vi "RunThis.vi"() -> ()   [LabVIEW 2017]
uses:
  states.ctl
  <vilib>/myRIO/Express VI/Onboard IO/DI/DI Express VI.xnode
  <vilib>/myRIO/Instrument Drivers/Onboard IO/DIO/typedefs/DIO Reference.ctl
  <vilib>/myRIO/Instrument Drivers/Onboard IO/DIO/DIO.lvlib
  <vilib>/myRIO/Common/Instrument Driver Framework/myRIO v1.0/DIO/typedefs/DIO Channels List.ctl
  <vilib>/myRIO/Common/Instrument Driver Framework/myRIO v1.0/DIO/typedefs/DIO Channels Enum.ctl
  <vilib>/myRIO/Common/Instrument Driver Framework/Utilities/typedefs/myRIO Generic Hardware Reference.ctl
  <vilib>/myRIO/Common/Instrument Driver Framework/Utilities/typedefs/myRIO v1.0 Reference.ctl
  <vilib>/myRIO/Common/Instrument Driver Framework/Utilities/typedefs/Generic FPGA Reference.ctl
  <vilib>/myRIO/Common/Instrument Driver Framework/Utilities/typedefs/Hardware Version Enum.ctl
  <vilib>/myRIO/Instrument Drivers/Onboard IO/DIO/vis/Read.vi
  <vilib>/myRIO/Instrument Drivers/Onboard IO/DIO/vis/myRIO DIO Open.xnode
  <vilib>/userdefined/High Color/nirio_resource_hc.ctl
  <vilib>/myRIO/Common/Instrument Driver Framework/myRIO v1.0/DIO/vis/myRIO v1.1 Open DIO.vi
  <vilib>/myRIO/Common/Instrument Driver Framework/Utilities/vis/Is FPGA Ref Available.vi
  encoderposition.ctl
  <vilib>/myRIO/Express VI/Onboard IO/DO/DO Express VI.xnode
  <vilib>/myRIO/Instrument Drivers/Onboard IO/DIO/vis/Write.vi
panel:
  in  "led ms":u32=25
  in  "Motor B":dbl
  out "ride mode duty cycle":dbl format="%.2f"
  out "rps (ride mode)":dbl
  out "Button 4":bool
  out "Counter Value":i32
  out "Button 1":bool
  out "Button 3":bool
  out "Button 2":bool
  in  "Stop Button":bool
  # "Control Panel"
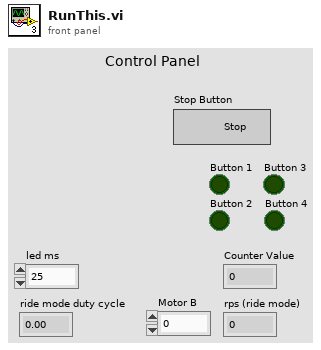
[diagram p1: front panel]
types:
  T1 = typedef "states.ctl" = enum16{"Calibration", "Button Debounce", "Reset Encoder", "Standby", "Go to Horse 1", "Go to Horse 2", "Go to Horse 3", "Go to Horse 4", "Ride Mode"}
  T2 = typedef "DIO.lvlib/DIO Reference.ctl" = cluster{"myRIO Reference":T3, "DIO Channels List":T7}
  T3 = typedef "myRIO Generic Hardware Reference.ctl" = cluster{"myRIO Model":T4, "myRIO Hardware Reference":T5}
  T4 = typedef "Hardware Version Enum.ctl" = enum16{"Unknown", "myRIO-1900", "myRIO-1950", "roboRIO", "NI ELVIS RIO CM"}
  T5 = typedef "myRIO v1.0 Reference.ctl" = cluster{"Generic FPGA Reference":T6, "Allow multiple opens":bool}
  T6 = typedef "Generic FPGA Reference.ctl" = refnum<k20>
  T7 = typedef "DIO Channels List.ctl" = T8[]
  T8 = typedef "DIO Channels Enum.ctl" = enum16{"Not Connected", "C/DIO0", "C/DIO1", "C/DIO2", "C/DIO3", "C/DIO4", "C/DIO5", "C/DIO6", "C/DIO7", "A/DIO0", "A/DIO1", "A/DIO2", "A/DIO3", "A/DIO4", "A/DIO5", "A/DIO6", "A/DIO7", "A/DIO8", "A/DIO9", "A/DIO10", "A/DIO11", "A/DIO12", "A/DIO13", "A/DIO14", "A/DIO15", "B/DIO0", "B/DIO1", "B/DIO2", "B/DIO3", "B/DIO4", "B/DIO5", "B/DIO6", "B/DIO7", "B/DIO8", "B/DIO9", "B/DIO10", "B/DIO11", "B/DIO12", "B/DIO13", "B/DIO14", "B/DIO15", "LED0", "LED1", "LED2", "LED3", "Button0", "DIO/DIO0", "DIO/DIO1", "DIO/DIO2", "DIO/DIO3", "DIO/DIO4", "DIO/DIO5", "DIO/DIO6", "DIO/DIO7", "DIO/DIO8", "DIO/DIO9", "SPI/CS0", "SPI/CS1", "SPI/CS2", "SPI/CS3", "LED RADIO (Green)", "LED RADIO (Red)", "LED COMM (Green)", "LED COMM (Red)", "LED MODE (Green)", "LED MODE (Red)"}
  T9 = typedef "nirio_resource_hc.ctl" = tag
  T10 = typedef "encoderposition.ctl" = u16
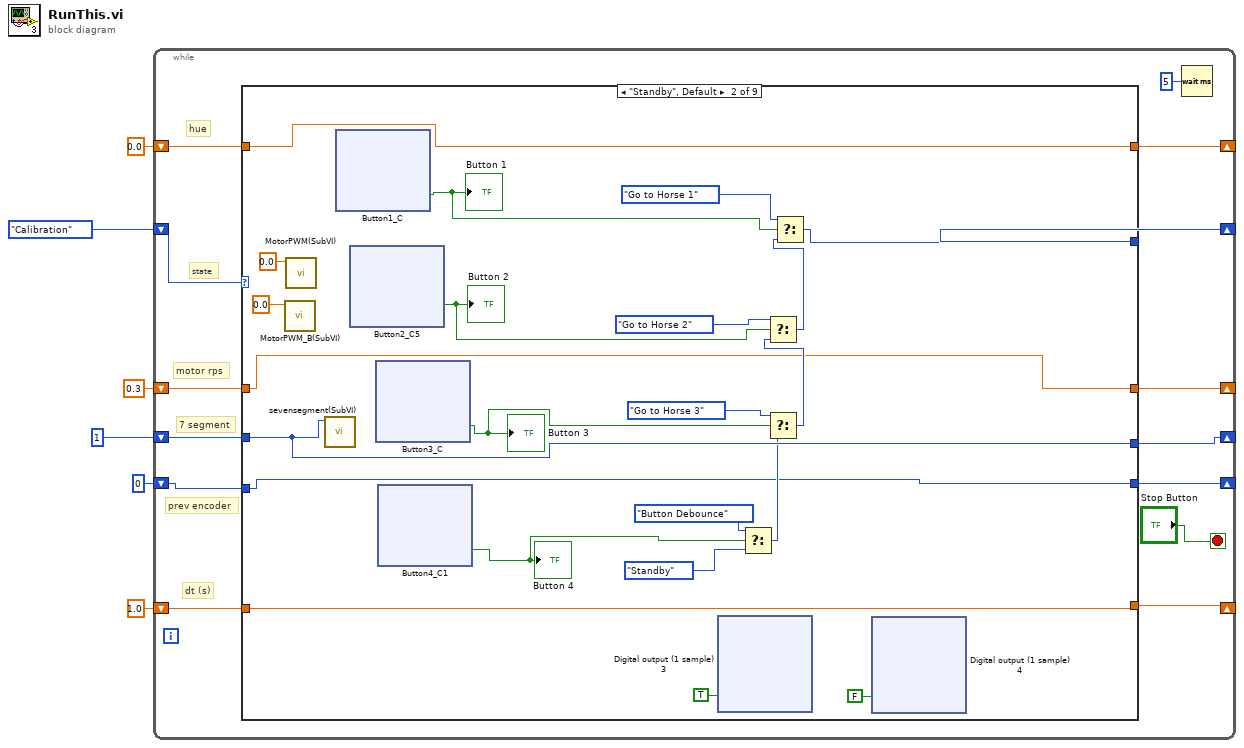
[diagram p0: block diagram]
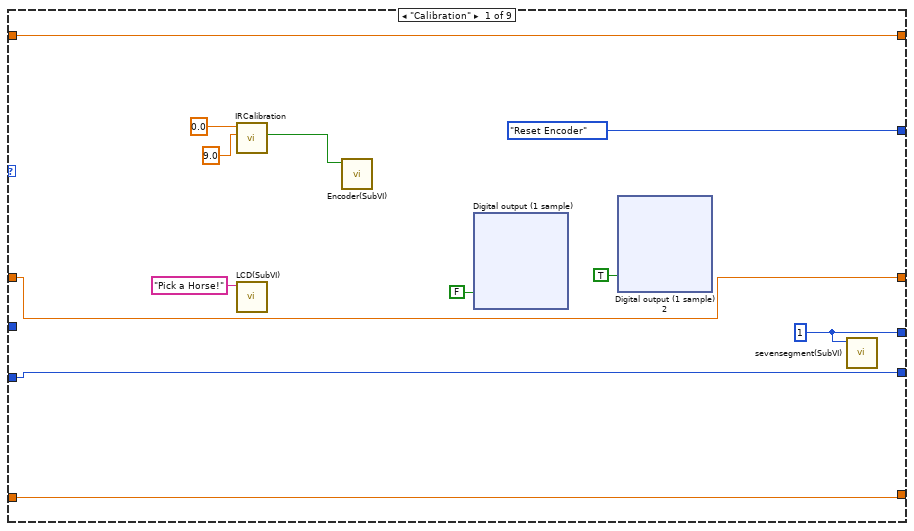
[diagram p2: hidden frame]
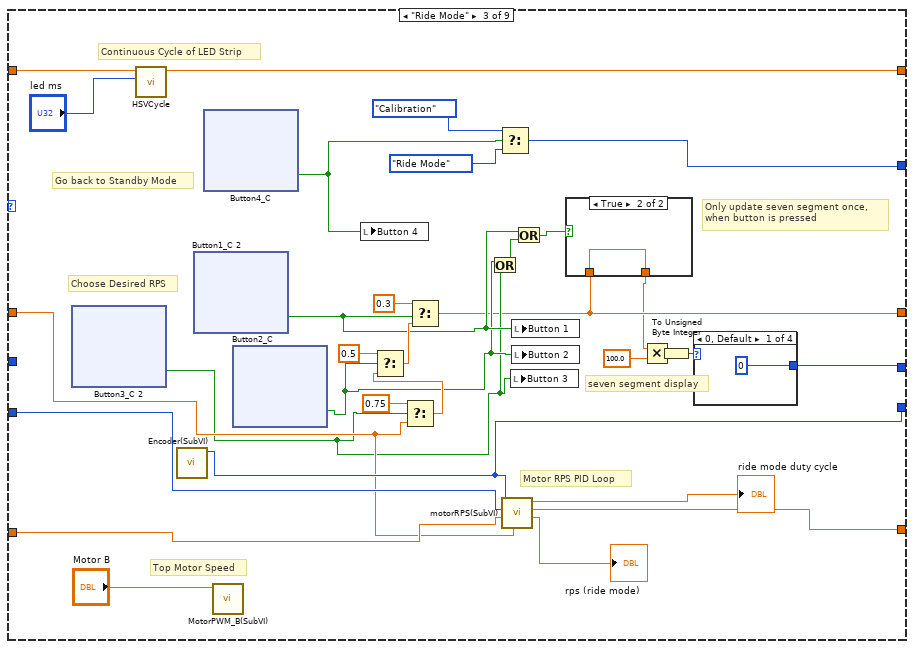
[diagram p3: hidden frame]
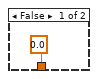
[diagram p4: hidden frame]
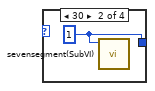
[diagram p5: hidden frame]
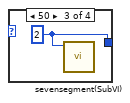
[diagram p6: hidden frame]
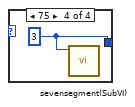
[diagram p7: hidden frame]
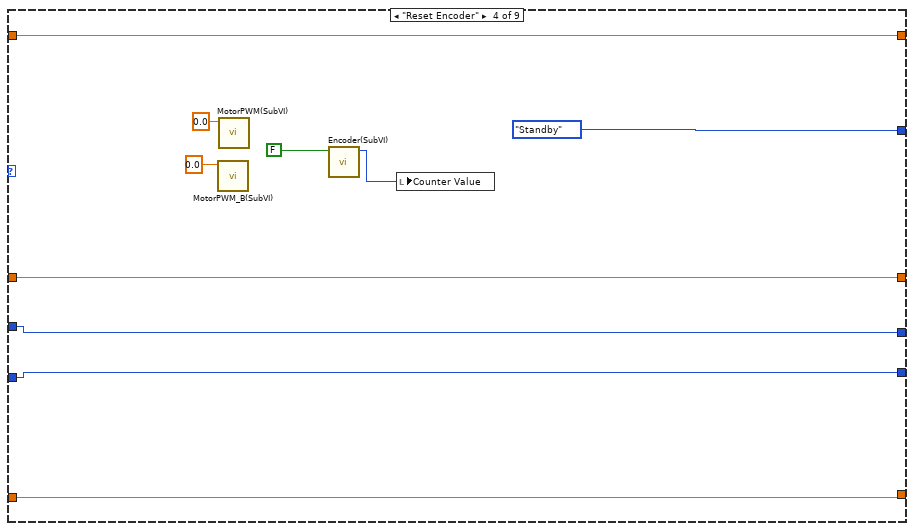
[diagram p8: hidden frame]
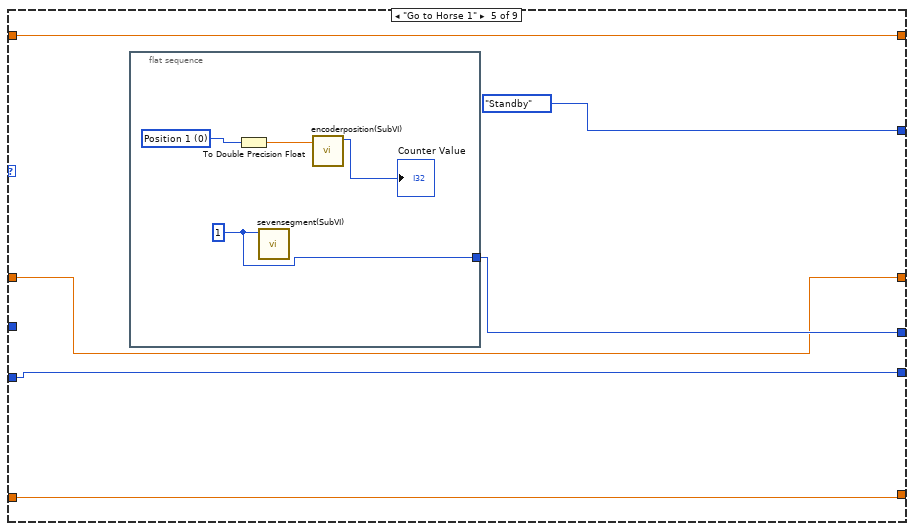
[diagram p9: hidden frame]
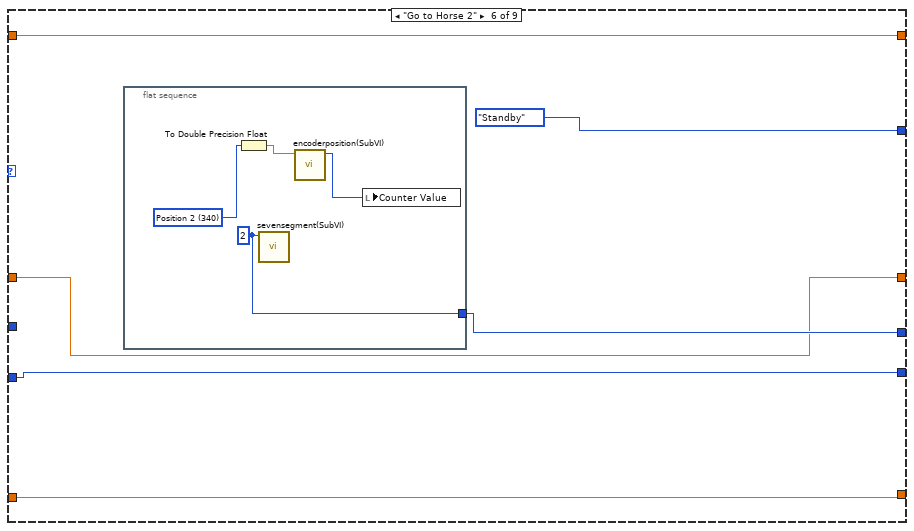
[diagram p10: hidden frame]
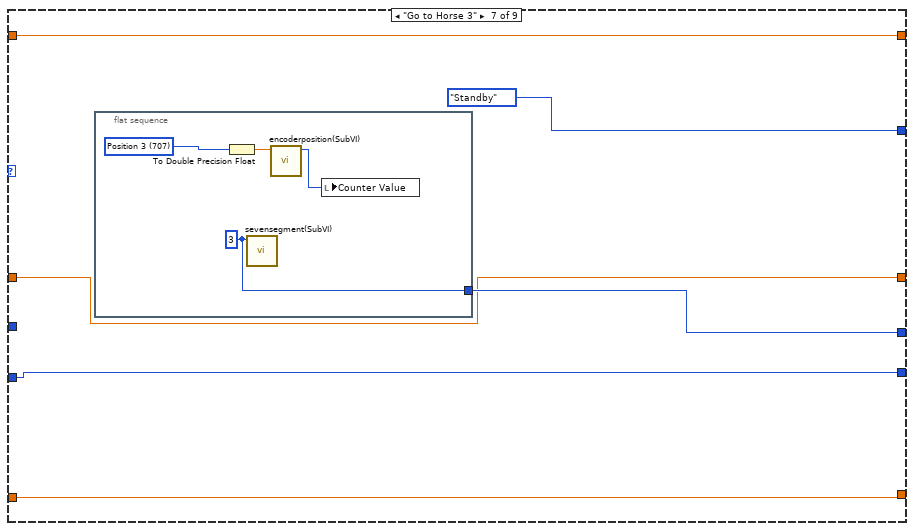
[diagram p11: hidden frame]
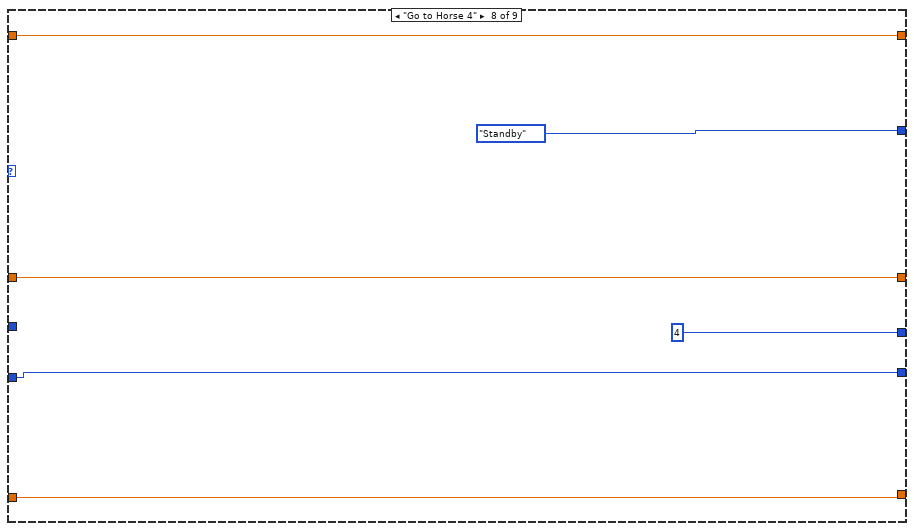
[diagram p12: hidden frame]
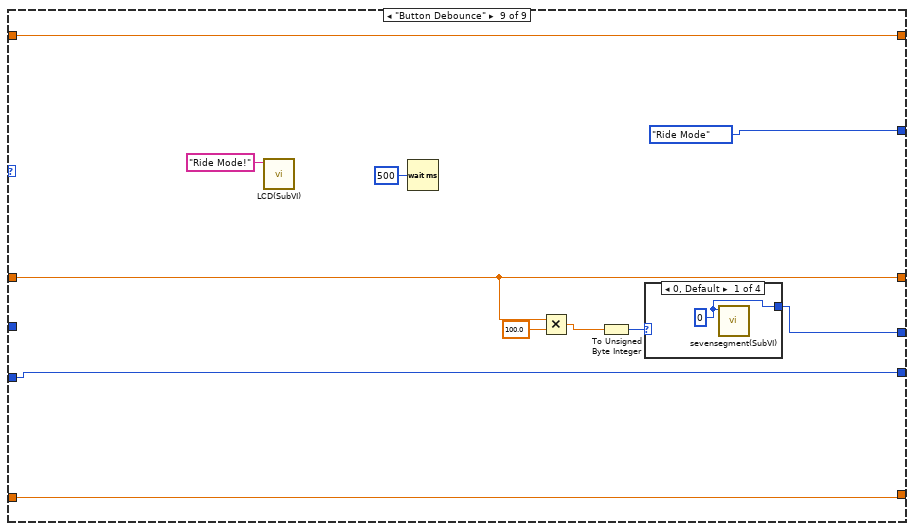
[diagram p13: hidden frame]
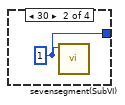
[diagram p14: hidden frame]
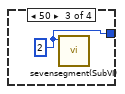
[diagram p15: hidden frame]
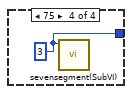
[diagram p16: hidden frame]
diagram:
  n1 = while {
    shift-right: [w19] -> _
    shift-left: states."Calibration" -> [w20]
    shift-right: [w15] -> _
    shift-left: 1 ("Numeric") -> [w16]
    shift-right: [w14] -> _
    shift-left: 0 ("Counter Value") -> [w13]
    shift-right: [w12] -> _
    shift-left: 1.0 ("dt out (s)") -> [w11]
    shift-right: [w10] -> _
    shift-left: 0.0 ("Hue Out") -> [w9]
    shift-right: [w8] -> _
    shift-left: 0.3 ("t") -> [w7]
    stop <- "Stop Button" stop-if-true
    # "motor rps"
    # "hue"
    # "state"
    # "dt (s)"
    # "prev encoder"
    # "7 segment"
    n2 = case shown="\"Standby\", Default" w20 {
      tunnel: [states."Reset Encoder" w121 w364 states."Standby" states."Standby" states."Standby" states."Standby" states."Standby" states."Ride Mode"] -> w19
      tunnel: w16 -> [_ w113 _ w516 _ _ _ _ _]
      tunnel: [w21 w113 w344 w516 w526 w536 w546 4 ("Numeric") w558] -> w15
      tunnel: [w27 w108 w361 w515 w525 w535 w545 w555 w568] -> w14
      tunnel: w13 -> [w27 w108 w362 w515 w525 w535 w545 w555 w568]
      tunnel: [w26 w107 w360 w514 w524 w534 w544 w554 w567] -> w12
      tunnel: w11 -> [w26 w107 w359 w514 w524 w534 w544 w554 w567]
      tunnel: [w25 w106 w355 w513 w523 w533 w543 w553 w566] -> w10
      tunnel: w9 -> [w25 w106 w354 w513 w523 w533 w543 w553 w566]
      tunnel: [w22 w103 w338 w512 w522 w532 w542 w552 w562] -> w8
      tunnel: w7 -> [w22 w103 w346 w512 w522 w532 w542 w552 w562]
      frame "Calibration" {
        w21 = 1 ("Numeric")
        n3 = call "IRCalibration.vi"("Stop Point"=9.0, "Duty Cycle (-100 to + 100)"=0.0) -> ("Boolean"=w32:bool)  [unwired: 8 in, 1 out]
        n4 = call "LCD(SubVI).vi"("String"="Pick a Horse!") -> ()  [unwired: 11 in]
        n5 = call "Encoder(SubVI).vi"("Reset Counter"=w32) -> ()  [unwired: 9 in, 2 out]
        n6 = xnode "Digital output (1 sample)"("LED_Green (A/DIO15 (Pin 34))"=FALSE) -> ()  [unwired: 1 in, 1 out]
        n7 = xnode "Digital output (1 sample) 2"("LED_Red (A/DIO14 (Pin 32))"=TRUE) -> ()  [unwired: 1 in, 1 out]
        n8 = call "sevensegment(SubVI).vi"("Numeric"=w21) -> ()  [unwired: 11 in]
      }
      frame "Standby", Default {
        n9 = call "MotorPWM_B(SubVI).vi"("Duty Cycle (-100 to + 100)"=0.0) -> ()  [unwired: 11 in]
        n10 = call "MotorPWM(SubVI).vi"("Duty Cycle (-100 to + 100)"=0.0) -> ()  [unwired: 11 in]
        n11 = call "sevensegment(SubVI).vi"("Numeric"=w113) -> ()  [unwired: 11 in]
        n12 = xnode "Button1_C"() -> ("C/DIO6 (DIO6)"=w124:bool)  [unwired: 1 in, 1 out]
        "Button 1" <- w124
        n13 = xnode "Button2_C5"() -> ("C/DIO5 (DIO5)"=w123:bool)  [unwired: 1 in, 1 out]
        "Button 2" <- w123
        n14 = xnode "Button3_C"() -> ("C/DIO4 (DIO4)"=w116:bool)  [unwired: 1 in, 1 out]
        "Button 3" <- w116
        n15 = xnode "Button4_C1"() -> ("C/DIO1 (DIO1)"=w111:bool)  [unwired: 1 in, 1 out]
        "Button 4" <- w111
        n16 = xnode "Digital output (1 sample) 3"("LED_Green (A/DIO15 (Pin 34))"=TRUE) -> ()  [unwired: 1 in, 1 out]
        n17 = Select(t=states."Button Debounce", s=w111, f=states."Standby") -> (s? t:f=w112:T1)
        n18 = Select(t=states."Go to Horse 3", s=w116, f=w112) -> (s? t:f=w118:T1)
        n19 = Select(t=states."Go to Horse 2", s=w123, f=w118) -> (s? t:f=w120:T1)
        n20 = Select(t=states."Go to Horse 1", s=w124, f=w120) -> (s? t:f=w121:T1)
        n21 = xnode "Digital output (1 sample) 4"("LED_Red (A/DIO14 (Pin 32))"=FALSE) -> ()  [unwired: 1 in, 1 out]
      }
      frame "Ride Mode" {
        # "Only update seven segment once, \nwhen button is pressed"
        # "Top Motor Speed"
        # "seven segment display"
        # "Choose Desired RPS"
        # "Motor RPS PID Loop"
        # "Continuous Cycle of LED Strip"
        # "Go back to Standby Mode"
        n22 = xnode "Button3_C 2"() -> ("C/DIO4 (DIO4)"=w339:bool)  [unwired: 1 in, 1 out]
        n23 = call "HSVCycle.vi"("milliseconds to wait"="led ms", "Hue"=w354) -> ("Hue Out"=w355:dbl)  [unwired: 9 in]
        n24 = call "Encoder(SubVI).vi"() -> ("Counter Value"=w361:i32)  [unwired: 10 in, 1 out]
        n25 = xnode "Button1_C 2"() -> ("C/DIO6 (DIO6)"=w341:bool)  [unwired: 1 in, 1 out]
        n26 = xnode "Button4_C"() -> ("C/DIO1 (DIO1)"=w353:bool)  [unwired: 1 in, 1 out]
        n27 = call "MotorPWM_B(SubVI).vi"("Duty Cycle (-100 to + 100)"="Motor B") -> ()  [unwired: 11 in]
        n28 = xnode "Button2_C"() -> ("C/DIO5 (DIO5)"=w340:bool)  [unwired: 1 in, 1 out]
        n29 = local write "Button 4"(w353) -> ()
        n30 = Select(t=0.75, s=w339, f=w346) -> (s? t:f=w348:dbl)
        n31 = Select(t=0.5, s=w340, f=w348) -> (s? t:f=w350:dbl)
        n32 = Select(t=0.3, s=w341, f=w350) -> (s? t:f=w338:dbl)
        n33 = Or(x=w340, y=w339) -> (x .or. y?=w342:bool)
        n34 = Select(t=states."Calibration", s=w353, f=states."Ride Mode") -> (s? t:f=w364:T1)
        n35 = call "motorRPS(SubVI).vi"("desired rps"=w346, "dt out (s) in"=w359, "Previous Encoder Value"=w362, "Current Encoder Value"=w361) -> ("rps (ride mode)"=→"rps (ride mode)":dbl, "dt out (s) out"=w360:dbl, "ride mode duty cycle"=→"ride mode duty cycle":dbl)  [unwired: 5 in]
        n36 = local write "Button 3"(w339) -> ()
        n37 = local write "Button 1"(w341) -> ()
        n38 = local write "Button 2"(w340) -> ()
        n39 = Or(x=w341, y=w342) -> (x .or. y?=w343:bool)
        n40 = case shown="True" w343 {
          tunnel: w338 -> [_ w367]
          tunnel: [0.0 ("t") w367] -> w337
          frame False {
          }
          frame True {
          }
        }
        n41 = Multiply(x=w337, y=100.0) -> (x*y=w336:dbl)
        n42 = To Unsigned Byte Integer(number=w336) -> (unsigned 8bit integer=w335:u8)
        n43 = case shown="0, Default" w335 {
          tunnel: [0 w369 w370 w371] -> w344
          frame 0, Default {
          }
          frame 30 {
            w369 = 1
            n44 = call "sevensegment(SubVI).vi"("Numeric"=w369) -> ()  [unwired: 11 in]
          }
          frame 50 {
            w370 = 2
            n45 = call "sevensegment(SubVI).vi"("Numeric"=w370) -> ()  [unwired: 11 in]
          }
          frame 75 {
            w371 = 3
            n46 = call "sevensegment(SubVI).vi"("Numeric"=w371) -> ()  [unwired: 11 in]
          }
        }
      }
      frame "Reset Encoder" {
        n47 = call "MotorPWM_B(SubVI).vi"("Duty Cycle (-100 to + 100)"=0.0) -> ()  [unwired: 11 in]
        n48 = call "MotorPWM(SubVI).vi"("Duty Cycle (-100 to + 100)"=0.0) -> ()  [unwired: 11 in]
        n49 = call "Encoder(SubVI).vi"("Reset Counter"=FALSE) -> ("Counter Value"=w517:i32)  [unwired: 9 in, 1 out]
        n50 = local write "Counter Value"(w517) -> ()
      }
      frame "Go to Horse 1" {
        n51 = flat-sequence {
          tunnel: [w530] -> w526
          frame #0 {
            w531 = T10 0 items=["Position 1"=0, "Position 2"=340, "Position 3"=707, "Position 4"=1080] ("Encoder Position")
            w530 = 1 ("Numeric")
            n52 = To Double Precision Float(number=w531) -> (double precision float=w529:dbl)
            n53 = call "sevensegment(SubVI).vi"("Numeric"=w530) -> ()  [unwired: 11 in]
            n54 = call "encoderposition(SubVI).vi"("Encoder Position"=w529) -> ("Counter Value"=→"Counter Value":i32)  [unwired: 9 in, 1 out]
          }
        }
      }
      frame "Go to Horse 2" {
        n55 = flat-sequence {
          tunnel: [w540] -> w536
          frame #0 {
            w541 = T10 340 items=["Position 1"=0, "Position 2"=340, "Position 3"=707, "Position 4"=1080] ("Encoder Position")
            w540 = 2 ("Numeric")
            n56 = To Double Precision Float(number=w541) -> (double precision float=w539:dbl)
            n57 = call "sevensegment(SubVI).vi"("Numeric"=w540) -> ()  [unwired: 11 in]
            n58 = call "encoderposition(SubVI).vi"("Encoder Position"=w539) -> ("Counter Value"=w538:i32)  [unwired: 9 in, 1 out]
            n59 = local write "Counter Value"(w538) -> ()
          }
        }
      }
      frame "Go to Horse 3" {
        n60 = flat-sequence {
          tunnel: [w551] -> w546
          frame #0 {
            w550 = T10 707 items=["Position 1"=0, "Position 2"=340, "Position 3"=707, "Position 4"=1080] ("Encoder Position")
            w551 = 3 ("Numeric")
            n61 = To Double Precision Float(number=w550) -> (double precision float=w549:dbl)
            n62 = call "sevensegment(SubVI).vi"("Numeric"=w551) -> ()  [unwired: 11 in]
            n63 = call "encoderposition(SubVI).vi"("Encoder Position"=w549) -> ("Counter Value"=w548:i32)  [unwired: 9 in, 1 out]
            n64 = local write "Counter Value"(w548) -> ()
          }
        }
      }
      frame "Go to Horse 4" {
      }
      frame "Button Debounce" {
        n65 = call "LCD(SubVI).vi"("String"="Ride Mode!") -> ()  [unwired: 11 in]
        n66 = Wait (ms)(milliseconds to wait=u32 500) -> ()  [unwired: 1 out]
        n67 = Multiply(x=w562, y=100.0) -> (x*y=w560:dbl)
        n68 = To Unsigned Byte Integer(number=w560) -> (unsigned 8bit integer=w559:u8)
        n69 = case shown="0, Default" w559 {
          tunnel: [w569 w570 w571 w572] -> w558
          frame 0, Default {
            w569 = 0
            n70 = call "sevensegment(SubVI).vi"("Numeric"=w569) -> ()  [unwired: 11 in]
          }
          frame 30 {
            w570 = 1
            n71 = call "sevensegment(SubVI).vi"("Numeric"=w570) -> ()  [unwired: 11 in]
          }
          frame 50 {
            w571 = 2
            n72 = call "sevensegment(SubVI).vi"("Numeric"=w571) -> ()  [unwired: 11 in]
          }
          frame 75 {
            w572 = 3
            n73 = call "sevensegment(SubVI).vi"("Numeric"=w572) -> ()  [unwired: 11 in]
          }
        }
      }
    }
    n74 = Wait (ms)(milliseconds to wait=u32 5) -> ()  [unwired: 1 out]
  }
